vi "MotorDriver.vi"(0 "Frequency [Hz]":dbl(slide)=1000.0 scale=0.0..1000.0, 5 "Duty Cycle in":dbl(slide)=0.5 scale=-1.0..1.0, 7 "Frequency [Hz] 2":dbl(slide)=1000.0 scale=0.0..1000.0, 9 "Duty Cycle in 2":dbl(slide)=0.5 scale=-1.0..1.0, 11 "error in (no error)":errorcluster) -> (4 "Duty Cycle out":dbl=0.5, 8 "Duty Cycle out 2":dbl=0.5, 15 "error out":errorcluster)   [LabVIEW 2019]
uses:
  <vilib>/myRIO/Instrument Drivers/Onboard IO/PWM/typedefs/PWM Reference.ctl
  <vilib>/myRIO/Common/Instrument Driver Framework/Utilities/typedefs/myRIO Generic Hardware Reference.ctl
  <vilib>/myRIO/Common/Instrument Driver Framework/Utilities/typedefs/Hardware Version Enum.ctl
  <vilib>/myRIO/Common/Instrument Driver Framework/Utilities/typedefs/myRIO v1.0 Reference.ctl
  <vilib>/myRIO/Common/Instrument Driver Framework/Utilities/typedefs/Generic FPGA Reference.ctl
  <vilib>/myRIO/Common/Instrument Driver Framework/myRIO v1.0/PWM/typedefs/PWM Channels Enum.ctl
  <vilib>/myRIO/Instrument Drivers/Onboard IO/PWM/typedefs/PWM Configuration.ctl
  <vilib>/userDefined/High Color/nirio_resource_hc.ctl
  <vilib>/myRIO/Instrument Drivers/Onboard IO/DIO/typedefs/DIO Reference.ctl
  <vilib>/myRIO/Common/Instrument Driver Framework/myRIO v1.0/DIO/typedefs/DIO Channels List.ctl
  <vilib>/myRIO/Common/Instrument Driver Framework/myRIO v1.0/DIO/typedefs/DIO Channels Enum.ctl
  <vilib>/myRIO/Common/Instrument Driver Framework/Utilities/vis/Is FPGA Ref Available.vi
  <vilib>/myRIO/Common/Instrument Driver Framework/myRIO v1.0/PWM/vis/myRIO v1.1 Open PWM.vi
  <vilib>/myRIO/Instrument Drivers/Onboard IO/PWM/vis/Set Duty Cycle and Frequency.vi
  <vilib>/myRIO/Common/Instrument Driver Framework/myRIO v1.0/DIO/vis/myRIO v1.1 Open DIO.vi
  <vilib>/myRIO/Instrument Drivers/Onboard IO/DIO/vis/Write.vi
  <vilib>/myRIO/Common/Instrument Driver Framework/Utilities/vis/Validate Channels.vi
  <vilib>/myRIO/Common/Instrument Driver Framework/myRIO v1.0/PWM/vis/myRIO v1.0 Reserve PWM.vi
  <vilib>/myRIO/Common/Instrument Driver Framework/myRIO v1.0/DIO/vis/myRIO v1.0 Reserve DIO.vi
  <vilib>/myRIO/Common/Instrument Driver Framework/myRIO v1.0/PWM/vis/myRIO v1.0 Build MUX Configuration PWM.vi
  <vilib>/myRIO/Common/Instrument Driver Framework/myRIO v1.0/Resource Manager/vis/myRIO v1.0 Reserve Channel List.vi
  <vilib>/myRIO/Common/Instrument Driver Framework/myRIO v1.0/DIO/vis/myRIO v1.0 Build MUX Configuration DIO.vi
  <vilib>/myRIO/Common/Instrument Driver Framework/myRIO v1.0/Resource Manager/vis/myRIO v1.0 Create Configuration List.vi
  <vilib>/myRIO/Common/Instrument Driver Framework/myRIO v1.0/Resource Manager/vis/myRIO v1.0 Reserve Channel.vi
  <vilib>/myRIO/Common/Instrument Driver Framework/myRIO v1.0/Resource Manager/vis/myRIO v1.0 Unreserve Channel.vi
  <vilib>/myRIO/Common/Instrument Driver Framework/myRIO v1.0/Resource Manager/vis/myRIO v1.0 Build Mutex Name.vi
  <vilib>/Utility/VariantDataType/GetNumericInfo.vi
  <vilib>/Utility/error.llb/Error Cluster From Error Code.vi
  <vilib>/myRIO/Common/Instrument Driver Framework/myRIO v1.0/myRIO v1.1 Open.vi
  <vilib>/myRIO/Common/Instrument Driver Framework/Utilities/vis/IO Manager.vi
  <vilib>/myRIO/Common/Instrument Driver Framework/Utilities/vis/Configuration Manager.vi
  <vilib>/myRIO/Common/Instrument Driver Framework/myRIO v1.0/Resource Manager/vis/myRIO v1.0 Configure IO.vi
  <vilib>/myRIO/Common/Instrument Driver Framework/myRIO v1.0/myRIO v1.0 Close.vi
  <vilib>/myRIO/Common/Instrument Driver Framework/myRIO v1.0/PWM/vis/myRIO v1.0 Write PWM.vi
  <vilib>/myRIO/Common/Instrument Driver Framework/myRIO v1.0/DIO/vis/myRIO v1.0 Write DIO.vi
  <vilib>/myRIO/Express VI/Onboard IO/PWM/PWM Express VI.xnode
  <vilib>/myRIO/Instrument Drivers/Onboard IO/PWM/vis/myRIO PWM Open.xnode
  <vilib>/myRIO/Express VI/Onboard IO/DO/DO Express VI.xnode
  <vilib>/myRIO/Instrument Drivers/Onboard IO/DIO/vis/myRIO DIO Open.xnode
  <vilib>/myRIO/Instrument Drivers/Onboard IO/PWM/PWM.lvlib
  <vilib>/myRIO/Instrument Drivers/Onboard IO/DIO/DIO.lvlib
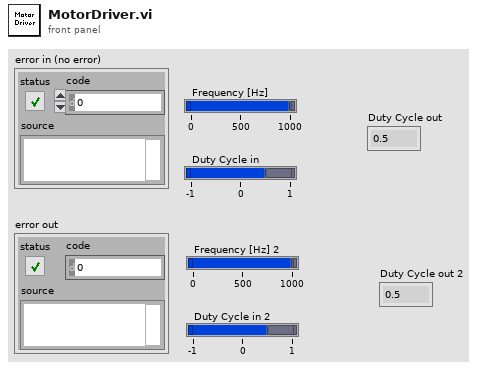
[diagram p1: front panel]
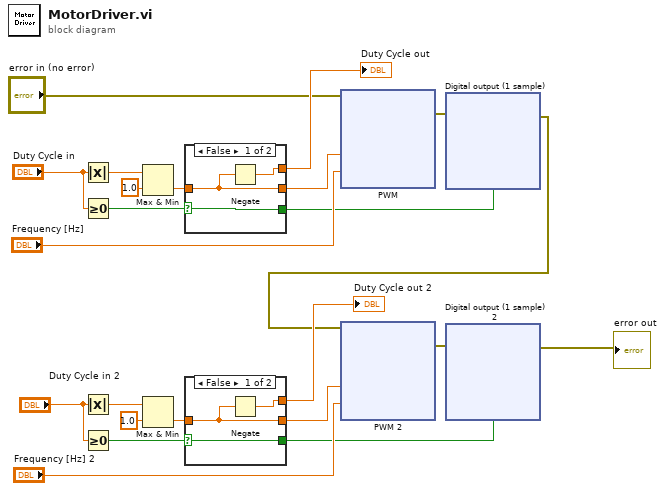
[diagram p0: block diagram]
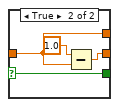
[diagram p2: hidden frame]
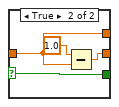
[diagram p3: hidden frame]
diagram:
  n1 = Absolute Value(x="Duty Cycle in") -> (abs(x)=w18:dbl)
  n2 = Greater Or Equal To 0?(x="Duty Cycle in") -> (x >= 0?=w19:bool)
  n3 = Absolute Value(x="Duty Cycle in 2") -> (abs(x)=w8:dbl)
  n4 = Greater Or Equal To 0?(x="Duty Cycle in 2") -> (x >= 0?=w9:bool)
  n5 = Max & Min(x=w18, y=1.0) -> (min(x,y)=w17:dbl)  [unwired: 1 out]
  n6 = Max & Min(x=w8, y=1.0) -> (min(x,y)=w7:dbl)  [unwired: 1 out]
  n7 = case shown="False" w19 {
    selector: w19 -> [w26 w28]
    tunnel: w17 -> [w25 w27]
    tunnel: [w25 w29] -> w16
    tunnel: [w26 w28] -> w14
    tunnel: [w24 w27] -> w15
    frame False {
      n8 = Negate(x=w25) -> (-x=w24:dbl)
    }
    frame True {
      n9 = Subtract(x=1.0, y=w27) -> (x-y=w29:dbl)
    }
  }
  "Duty Cycle out" <- w15
  n10 = case shown="False" w9 {
    selector: w9 -> [w33 w35]
    tunnel: w7 -> [w32 w34]
    tunnel: [w32 w36] -> w6
    tunnel: [w33 w35] -> w1
    tunnel: [w31 w34] -> w5
    frame False {
      n11 = Negate(x=w32) -> (-x=w31:dbl)
    }
    frame True {
      n12 = Subtract(x=1.0, y=w34) -> (x-y=w36:dbl)
    }
  }
  "Duty Cycle out 2" <- w5
  n13 = xnode "PWM"("Duty Cycle"=w16, "Frequency [Hz]"="Frequency [Hz]", "error in (no error)"="error in (no error)") -> ("error out"=w23:errorcluster)
  n14 = xnode "Digital output (1 sample)"("C/DIO5 (DIO5)"=w14, "error in (no error)"=w23) -> ("error out"=w3:errorcluster)
  n15 = xnode "PWM 2"("Duty Cycle"=w6, "Frequency [Hz]"="Frequency [Hz] 2", "error in (no error)"=w3) -> ("error out"=w13:errorcluster)
  n16 = xnode "Digital output (1 sample) 2"("C/DIO1 (DIO1)"=w1, "error in (no error)"=w13) -> ("error out"=→"error out":errorcluster)
